vi "Test Cryo-Con.vi"() -> ()   [LabVIEW 2021]
uses:
  Temperature Controller Driver/T controller configuration.ctl
  Temperature Controller/Controls/Control Mode.ctl
  Cryo-Con Driver/Cryo-Con Driver.lvclass
  C:/GitHub/NHMFL_Core/Libraries/Instruments/Temperature Controller Driver/Temperature Controller Driver.lvclass
  C:/GitHub/NHMFL_Core/Libraries/Instruments/Instrument Driver/Instrument Driver.lvclass
  C:/GitHub/NHMFL_Core/Libraries/Instruments/VISA Instrument/VISA Instrument.lvclass
  LabActor/Instrument Actor/Instrument Actor.lvclass/Instrument Actor.ctl
  VISA Instrument/VISA Instrument.lvclass/VISA Instrument.ctl
  LabActor/Instrument Actor/Read Instrument driver.vi
  VISA Instrument/Read VISA resource.vi
  Temperature Controller Driver/Write T controller configuration.vi
  Instrument Driver/Write User configuration.vi
  Instrument Driver/Instrument Driver.lvclass
  LabActor/Instrument Actor/Instrument Actor.lvclass
panel:
  out "read buffer":string
  in  "Refresh from instrument":bool
  in  "Configuration":T1={"Record Channels"=["A"], "Record raw signal"=FALSE, "Set point"=0.0, "Record heater"=FALSE, "Ramp rate"=0.0, "P"=0.0, "I"=0.0, "D"=0.0, "Control"=enum."Off", "P manual"=0.0, "Output #"=1}
  in  "Stop Button":bool
  out "Temperature":dbl format="%.5f"
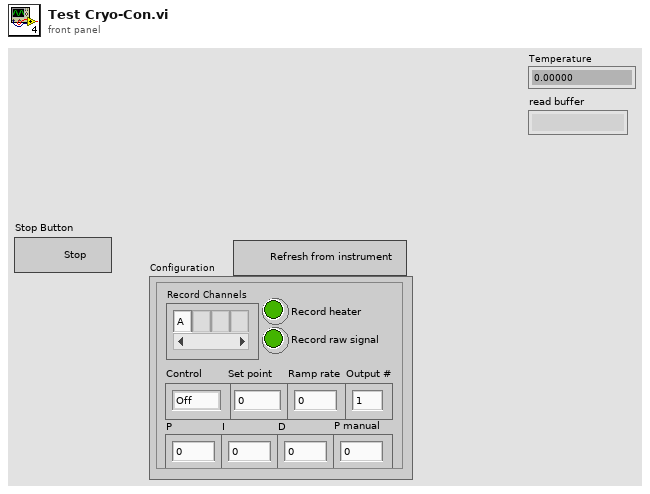
[diagram p1: front panel]
types:
  T1 = typedef "T controller configuration.ctl" = cluster{"Record Channels":string[], "Record raw signal":bool, "Set point":dbl, "Record heater":bool, "Ramp rate":dbl, "P":dbl, "I":dbl, "D":dbl, "Control":T2, "P manual":dbl, "Output #":i32}
  T2 = typedef "Control Mode.ctl" = enum16{"Off", "PID", "Ramp", "Manual", "Table"}
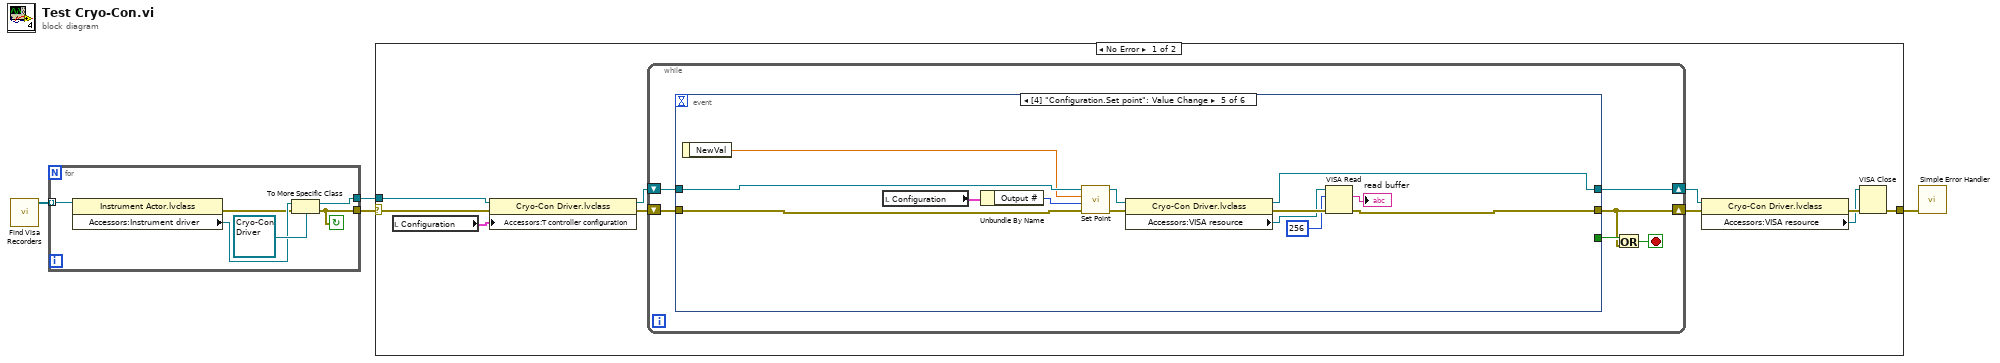
[diagram p0: block diagram]
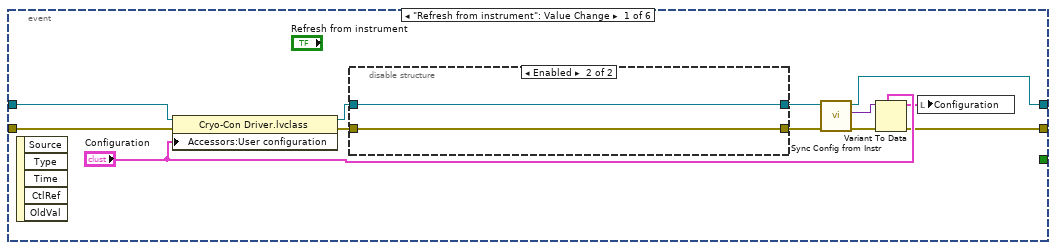
[diagram p2: hidden frame]
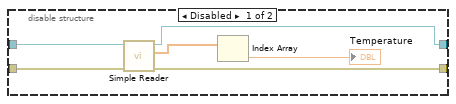
[diagram p3: hidden frame]
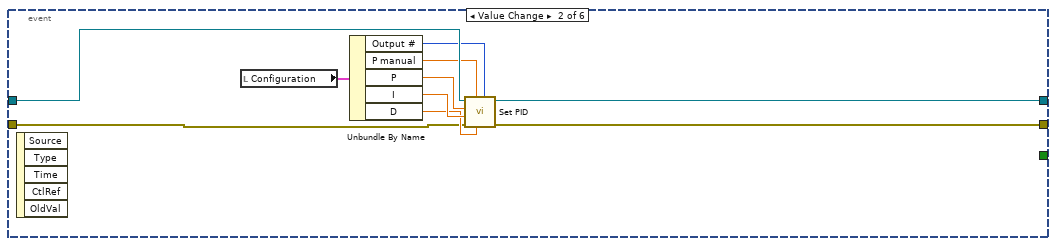
[diagram p4: hidden frame]
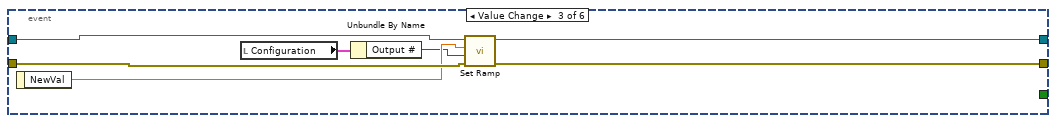
[diagram p5: hidden frame]
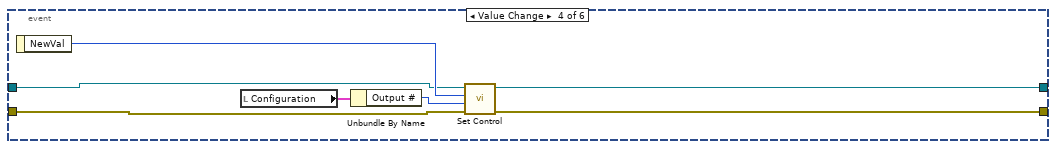
[diagram p6: hidden frame]
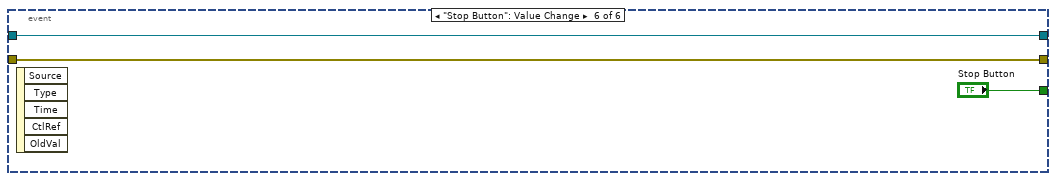
[diagram p7: hidden frame]
diagram:
  n1 = call "Find Visa Recorders.vi"() -> ("Recorders List"=w3:refnum<class "Instrument Actor.lvclass">[])  [unwired: 9 in, 2 out]
  n2 = for {
    tunnel: w3 -> [w10] mode=indexing
    tunnel: [w8] -> w1
    tunnel: [w7] -> w2
    stop <- w8 continue-if-true
    n3 = property class="Instrument Actor.lvclass"(reference=w10) -> (error out=w5:errorcluster, "Accessors:Instrument driver"=w6:refnum<class "Instrument Driver.lvclass">)  [unwired: 1 in, 1 out]
    n4 = To More Specific Class(target class=refnum<class "Cryo-Con Driver.lvclass"> refnum ("Cryo-Con Driver.lvclass"), reference=w6, error in=w5) -> (specific class reference=w7:refnum<class "Cryo-Con Driver.lvclass">, error out=w8:errorcluster)
  }
  n5 = case shown="No Error" w1 {
    selector: w1 -> [w11 w87]
    tunnel: [w20 w87] -> w4
    tunnel: w2 -> [w12 _]
    frame No Error {
      n6 = local read "Configuration"() -> (w13:T1)
      n7 = property class="Cryo-Con Driver.lvclass"(reference=w12, error in=w11, "Accessors:T controller configuration"=w13) -> (reference out=w19:refnum<class "Cryo-Con Driver.lvclass">, error out=w18:errorcluster)
      n8 = while {
        shift-right: [w23] -> w14
        shift-left: w18 -> [w26]
        shift-right: [w21] -> w17
        shift-left: w19 -> [w22]
        stop <- w24 stop-if-true
        n9 = event shown="[4] \"Configuration.Set point\": Value Change" {
          selector: _ -> [_ _ _ _ _ _]
          dyn-events: _ -> [_ _ _ _ _ _]
          timeout: _ -> [_ _ _ _ _ _]
          tunnel: w26 -> [w27 w49 w62 w68 w82 w85]
          tunnel: [w33 w50 w61 w69 w72 w85] -> w23
          tunnel: [_ _ _ _ _ "Stop Button"] -> w25
          tunnel: w22 -> [w31 w56 w63 w66 w83 w84]
          tunnel: [w38 w51 w60 w67 w76 w84] -> w21
          event "Refresh from instrument": Value Change {
            n10 = event-data() -> ()  [unwired: 1 in, 5 out]
            n11 = property class="Cryo-Con Driver.lvclass"(reference=w31, error in=w27, "Accessors:User configuration"="Configuration") -> (reference out=w30:refnum<class "Cryo-Con Driver.lvclass">, error out=w32:errorcluster)
            n12 = disable-structure shown="Enabled" {
              disable-tunnel: w32 -> [w42 w45]
              disable-tunnel: w30 -> [w41 w46]
              disable-tunnel: [w40 w46] -> w29
              disable-tunnel: [w39 w45] -> w28
              frame Disabled {
                n13 = call-dynamic "Simple Reader.vi"("error in (no error)"=w42, "Cryo-Con Driver in"=w41) -> ("error out"=w39:errorcluster, "Signals"=w44:dbl[], "Cryo-Con Driver out"=w40:refnum<class "Cryo-Con Driver.lvclass">)  [unwired: 7 in]
                n14 = Index Array(array=w44) -> (element=→"Temperature":dbl)  [unwired: 1 in]
              }
              frame Enabled {
              }
            }
            n15 = call-dynamic "Sync Config from Instr.vi"("error in (no error)"=w28, "Cryo-Con Driver in"=w29) -> ("error out"=w37:errorcluster, "Variant"=w36:variant, "Cryo-Con Driver out"=w38:refnum<class "Cryo-Con Driver.lvclass">)  [unwired: 7 in]
            n16 = Variant To Data(error in=w37, type="Configuration", Variant=w36) -> (data=w34:T1, error out=w33:errorcluster)
            n17 = local write "Configuration"(w34) -> ()
          }
          event Value Change {
            n18 = event-data() -> ()  [unwired: 1 in, 5 out]
            n19 = local read "Configuration"() -> (w55:T1)
            n20 = Unbundle By Name(w55) -> ("Output #"=w47:i32, "P manual"=w48:dbl, "P"=w54:dbl, "I"=w53:dbl, "D"=w52:dbl)
            n21 = call-dynamic "Set PID.vi"("Output #"=w47, "D"=w52, "P manual"=w48, "error in (no error)"=w49, "I"=w53, "P"=w54, "Cryo-Con Driver in"=w56) -> ("error out"=w50:errorcluster, "Cryo-Con Driver out"=w51:refnum<class "Cryo-Con Driver.lvclass">)  [unwired: 3 in]
          }
          event Value Change {
            n22 = event-data() -> ("NewVal"=w59:dbl)  [unwired: 1 in]
            n23 = local read "Configuration"() -> (w58:T1)
            n24 = Unbundle By Name(w58) -> ("Output #"=w57:i32)
            n25 = call-dynamic "Set Ramp.vi"("error in (no error)"=w62, "Output #"=w57, "Ramp rate (0: off)"=w59, "Cryo-Con Driver in"=w63) -> ("error out"=w61:errorcluster, "Cryo-Con Driver out"=w60:refnum<class "Cryo-Con Driver.lvclass">)  [unwired: 6 in]
          }
          event Value Change {
            n26 = event-data() -> ("NewVal"=w70:T2)  [unwired: 1 in]
            n27 = local read "Configuration"() -> (w65:T1)
            n28 = Unbundle By Name(w65) -> ("Output #"=w64:i32)
            n29 = call-dynamic "Set Control.vi"("error in (no error)"=w68, "Output #"=w64, "Control"=w70, "Cryo-Con Driver in"=w66) -> ("error out"=w69:errorcluster, "Cryo-Con Driver out"=w67:refnum<class "Cryo-Con Driver.lvclass">)  [unwired: 6 in]
          }
          event Value Change {
            n30 = event-data() -> ("NewVal"=w80:dbl)  [unwired: 1 in]
            n31 = local read "Configuration"() -> (w79:T1)
            n32 = Unbundle By Name(w79) -> ("Output #"=w78:i32)
            n33 = call-dynamic "Set Point.vi"("error in (no error)"=w82, "Output #"=w78, "Set point"=w80, "Cryo-Con Driver in"=w83) -> ("error out"=w81:errorcluster, "Cryo-Con Driver out"=w77:refnum<class "Cryo-Con Driver.lvclass">)  [unwired: 6 in]
            n34 = property class="Cryo-Con Driver.lvclass"(reference=w77, error in=w81) -> (reference out=w76:refnum<class "Cryo-Con Driver.lvclass">, error out=w75:errorcluster, "Accessors:VISA resource"=w74:refnum<visa-resource-name>)
            n35 = VISA Read(VISA resource name=w74, byte count=u32 256, error in (no error)=w75) -> (read buffer=→"read buffer":string, error out=w72:errorcluster)  [unwired: 2 out]
          }
          event "Stop Button": Value Change {
            n36 = event-data() -> ()  [unwired: 1 in, 5 out]
          }
        }
        n37 = Or(x=w25, y=w23) -> (x .or. y?=w24:bool)
      }
      n38 = property class="Cryo-Con Driver.lvclass"(reference=w17, error in=w14) -> (error out=w16:errorcluster, "Accessors:VISA resource"=w15:refnum<visa-resource-name>)  [unwired: 1 out]
      n39 = VISA Close(VISA resource name=w15, error in (no error)=w16) -> (error out=w20:errorcluster)
    }
    frame Error {
    }
  }
  n40 = call <vilib>:"Simple Error Handler.vi"("error in (no error)"=w4) -> ()  [unwired: 4 in, 5 out]
